vi "PH_Cont-601k_PowerUnit.destructor.vi"(0 "i ref in":refnum<vi>, 5 "error in(no error)":errorcluster) -> (19 "error out":errorcluster)   [LabVIEW 2014, in "PH_Cont-601k_PowerUnit.lvlib"]
doc: "This is the destructor of a class.\n\nLicense Agreement for this software:\n\nCopyright (C)\nGesellschaft für Schwerionenforschung, GSI\nPlanckstr. 1\n64291 Darmstadt\nGermany\n\nContact: D.Beck@gsi.de \n\nThis program is free software; you can redistribute it and/or modify it under the terms of the \nGNU General Public License as published by the Free Software Foundation; either version 2 of \nthe license, or (at your option) any later version.\n\nThis program is distributed in the hope that it will be useful, but WITHOUT ANY WARRANTY; \nwithout even the implied warranty of MERCHANTABILITY or FITNESS FOR A PARTICULAR PURPOSE. See the GNU General License for more details (http://www.gnu.org).\n\nGesellschaft für Schwerionenforschung, GSI\nPlanckstr. 1, 64291 Darmstadt, Germany\nFor all questions and ideas contact: M.Richter@gsi.de, H.Brand@gsi.de or D.Beck@gsi.de.\nLast update: 16-JUN-2004"
uses:
  PH_Cont-601k_PowerUnit.lvlib
  PH_Cont-601k_PSU/PH_Cont-601k_PSU.lvlib
  lib.lib/DimLVEvent/LVDimInterface/LVDimInterface.lvlib
  PH_PowerUnit_BaseClass/PH_PowerUnit_BaseClass.lvlib
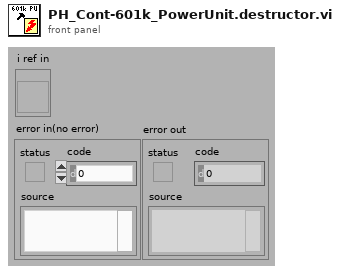
[diagram p1: front panel]
types:
  T1 = enum16{"SetAttribute", "GetAttribute", "CreateAttribute", "DestroyAttribute", "DestroyAllAtributes"}
  T2 = typedef "PH_Cont-601k_PowerUnit.lvlib/PH_Cont-601k_PowerUnit.i attribute.ctl" = cluster{"Service ID Last Shot":i32}
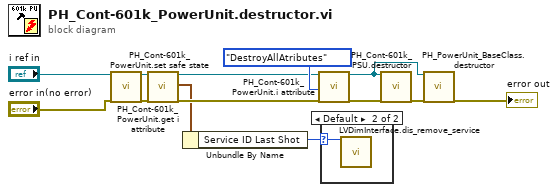
[diagram p0: block diagram]
diagram:
  n1 = call "PH_Cont-601k_PowerUnit.set safe state.vi"("i ref in"="i ref in", "error in (no error)"="error in(no error)") -> ("i ref out"=w3:refnum<vi>, "error out"=w5:errorcluster)  [unwired: 16 in]
  n2 = call "PH_Cont-601k_PowerUnit.get i attribute.vi"("i ref in"=w3, "error in (no error)"=w5) -> ("i ref out"=w11:refnum<vi>, "i attribute"=w10:T2, "error out"=w12:errorcluster)  [unwired: 15 in]
  n3 = Unbundle By Name(w10) -> ("Service ID Last Shot"=w9:i32)
  n4 = call "PH_Cont-601k_PowerUnit.i attribute.vi"("VI Refnum"=w11, "Action"=T1."DestroyAllAtributes", "error in (no error)"=w12) -> ("VI Refnum out"=w2:refnum<vi>, "error out"=w7:errorcluster)  [unwired: 14 in, 1 out]
  n5 = case shown="Default" w9 {
    selector: w9 -> [_ w14]
    frame -1 {
    }
    frame Default {
      n6 = call "LVDimInterface.dis_remove_service.vi"("my_serviceID"=w14) -> ()  [unwired: 18 in, 1 out]
    }
  }
  n7 = call "PH_Cont-601k_PSU.destructor.vi"("i ref in"=w2, "error in(no error)"=w7) -> ("error out"=w6:errorcluster)  [unwired: 17 in]
  n8 = call "PH_PowerUnit_BaseClass.destructor.vi"("i ref in"=w2, "error in(no error)"=w6) -> ("error out"=→"error out":errorcluster)  [unwired: 17 in]
